vi "Update.vi"(8 "error in":errorcluster, 11 "cCRD Subject in":refnum<class "cCRD Subject.lvclass">) -> (0 "error out":errorcluster, 2 "Stop?":bool, 3 "cCRD Subject out":refnum<class "cCRD Subject.lvclass">)   [LabVIEW 2015, in "cCRD Subject.lvclass"]
doc: "Default action of the Update function is strictly to see if a stop execution has been sent."
uses:
  cCRD Subject.lvclass
  Reusable/Data/Data.lvclass
  CRDS/Data/cCRDS Data.lvclass
  Reusable/Observer/Data Subject.lvclass/Data Subject.ctl
  Reusable/Observer/Accessors/Read Observer Refs.vi
  Reusable/Observer/Accessors/Read DVR.vi
  Reusable/Observer/Data Subject.lvclass
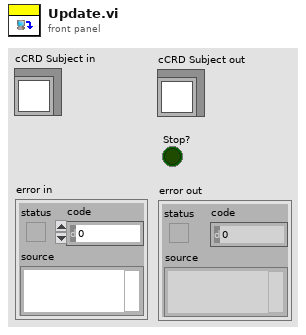
[diagram p1: front panel]
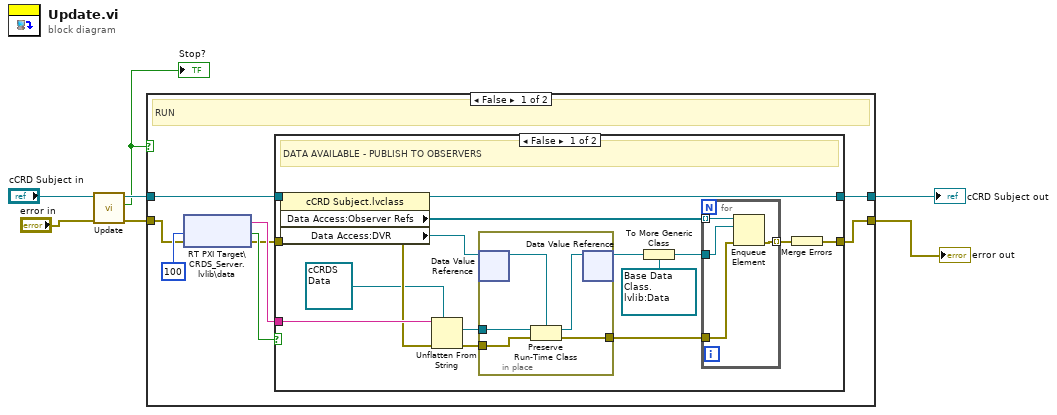
[diagram p0: block diagram]
diagram:
  n1 = call-parent "Update.vi"("error in"="error in", "Data Subject in"="cCRD Subject in") -> ("error out"=w6:errorcluster, "Stop?"=w5:bool, "Data Subject out"=w7:refnum<class "cCRD Subject.lvclass">)  [unwired: 7 in]
  "Stop?" <- w5
  n2 = case shown="False" w5 {
    tunnel: w7 -> [w12 w44]
    tunnel: [w11 w44] -> w2
    tunnel: [w9 w43] -> w1
    tunnel: w6 -> [w8 w43]
    frame False {
      # "RUN"
      n3 = shared-variable "RT PXI Target\\CRDS_Server.lvlib\\data"(error in=w8, 100 ("ms timeout (0)")) -> (w14:string, error out=w10:errorcluster, w13:bool)
      n4 = case shown="False" w13 {
        tunnel: w14 -> [w28 _]
        tunnel: w12 -> [w27 w42]
        tunnel: [w24 w42] -> w11
        tunnel: w10 -> [w23 w41]
        tunnel: [w18 w41] -> w9
        frame False {
          # "DATA AVAILABLE - PUBLISH TO OBSERVERS"
          n5 = property class="cCRD Subject.lvclass"(reference=w27, error in=w23) -> (reference out=w24:refnum<class "cCRD Subject.lvclass">, error out=w19:errorcluster, "Data Access:Observer Refs"=w26:refnum<queue>[], "Data Access:DVR"=w25:refnum<data-value>)
          n6 = Unflatten From String(type=refnum<class "cCRDS Data.lvclass"> refnum ("cCRDS Data"), binary string=w28, error in (no error)=w19) -> (value=w29:refnum<class "cCRDS Data.lvclass">, error out=w21:errorcluster)  [unwired: 2 in, 1 out]
          n7 = in-place {
            in-place-border: w29 -> [w40]
            in-place-border: [w37] -> w20
            in-place-border: w21 -> [w36]
            n8 = in-place-dvr #1(w25) -> (w39:refnum<class "Data.lvclass">)  [unwired: 1 out]
            n9 = Preserve Run-Time Class(object in=w40, error in=w36, 2:w39) -> (object out=w38:refnum<class "Data.lvclass">, error out=w37:errorcluster)
            n10 = in-place-dvr #1(w38) -> (w31:refnum<data-value>)  [unwired: 1 out]
          }
          n11 = To More Generic Class(target class=refnum<data-value> refnum ("data value reference"), reference=w31) -> (generic class reference=w30:refnum<data-value>)
          n12 = for {
            tunnel: w30 -> [w35]
            tunnel: w26 -> [w34] mode=indexing
            tunnel: w20 -> [w33]
            tunnel: [w32] -> w17 mode=indexing
            n13 = Enqueue Element(queue=w34, element=w35, error in (no error)=w33) -> (error out=w32:errorcluster)  [unwired: 1 in, 2 out]
          }
          n14 = Merge Errors(w17) -> (w18:errorcluster)
        }
        frame True {
          # "NO DATA AVAILABLE"
        }
      }
    }
    frame True {
      # "STOP"
    }
  }
  "error out" <- w1
  "cCRD Subject out" <- w2
